vi "Initialize Andor.vi"() -> ()   [LabVIEW 2014]
uses:
  SubVIs/Initilize Globals.vi
  lib/Andorlib/atmcd32d.lvlib
panel:
  out "HS Speed":dbl format="%#_13g"
  out "Number HS Speeds":i32
  out "VS Speed":dbl format="%#_13g"
  out "Number VS Speeds":i32
  out "Camera FirmWare Version":i32
  out "Y-pixels":i32
  out "X-pixels":i32
  out "Error Out 2":errorcluster
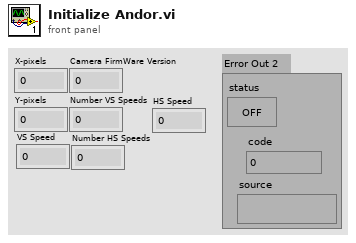
[diagram p1: front panel]
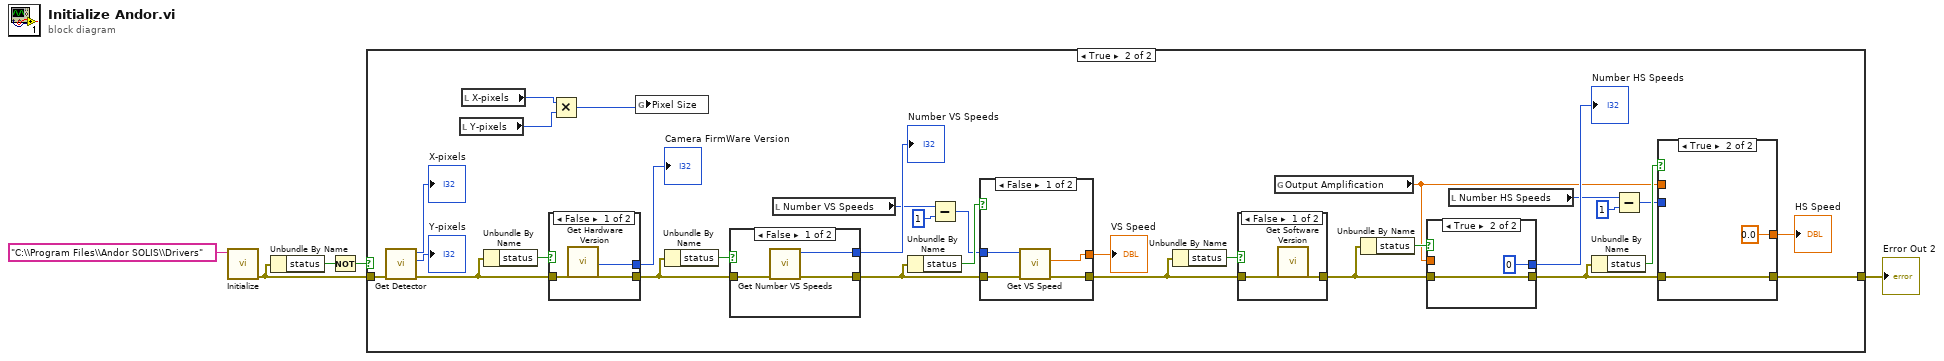
[diagram p0: block diagram]
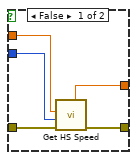
[diagram p3: hidden frame]
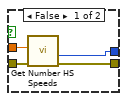
[diagram p4: hidden frame]
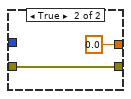
[diagram p6: hidden frame]
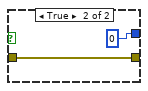
[diagram p7: hidden frame]
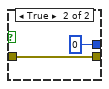
[diagram p8: hidden frame]
diagram:
  n1 = call "Initialize.vi"("dir"="C:\\Program Files\\Andor SOLIS\\Drivers") -> ("error out"=w2:errorcluster)  [unwired: 8 in, 2 out]
  n2 = Unbundle By Name(w2) -> ("status"=w5:bool)
  n3 = Not(x=w5) -> (.not. x?=w4:bool)
  n4 = case shown="True" w4 {
    tunnel: [w6 w25] -> w3
    tunnel: w2 -> [w6 w37]
    frame False {
    }
    frame True {
      n5 = call "Get Detector.vi"("error in (no error)"=w37) -> ("error out"=w30:errorcluster, "ypixels out"=→"Y-pixels":i32, "xpixels out"=→"X-pixels":i32)  [unwired: 7 in, 1 out]
      n6 = local read "Y-pixels"() -> (w8:i32)
      n7 = local read "X-pixels"() -> (w9:i32)
      n8 = Unbundle By Name(w30) -> ("status"=w36:bool)
      n9 = case shown="False" w36 {
        tunnel: w30 -> [w67 w69]
        tunnel: [w66 w69] -> w29
        tunnel: [w65 0] -> w21
        frame False {
          n10 = call "Get Hardware Version.vi"("error in (no error)"=w67) -> ("CameraFirmwareVersion out"=w65:u32, "error out"=w66:errorcluster)  [unwired: 19 in, 6 out]
        }
        frame True {
        }
      }
      "Camera FirmWare Version" <- w21
      n11 = Multiply(x=w9, y=w8) -> (x*y=w7:i32)
      n12 = global write "Initilize Globals.vi" "Pixel Size"(w7) -> ()
      n13 = Unbundle By Name(w29) -> ("status"=w35:bool)
      n14 = case shown="False" w35 {
        tunnel: w29 -> [w62 w64]
        tunnel: [w61 w64] -> w28
        tunnel: [w60 0] -> w20
        frame False {
          n15 = call "Get Number VS Speeds.vi"("error in (no error)"=w62) -> ("error out"=w61:errorcluster, "speeds out"=w60:i32)  [unwired: 8 in, 1 out]
        }
        frame True {
        }
      }
      "Number VS Speeds" <- w20
      n16 = local read "Number VS Speeds"() -> (w19:i32)
      n17 = Unbundle By Name(w28) -> ("status"=w34:bool)
      n18 = Subtract(x=w19, y=1) -> (x-y=w17:i32)
      n19 = case shown="False" w34 {
        tunnel: w28 -> [w56 w59]
        tunnel: [w57 w59] -> w27
        tunnel: w17 -> [w55 _]
        tunnel: [w54 0.0] -> w16
        frame False {
          n20 = call "Get VS Speed.vi"("error in (no error)"=w56, "index"=w55) -> ("error out"=w57:errorcluster, "speed out"=w54:sgl)  [unwired: 7 in, 1 out]
        }
        frame True {
        }
      }
      "VS Speed" <- w16
      n21 = Unbundle By Name(w27) -> ("status"=w33:bool)
      n22 = case shown="False" w33 {
        tunnel: w27 -> [w52 w53]
        tunnel: [w51 w53] -> w26
        frame False {
          n23 = call "Get Software Version.vi"("error in (no error)"=w52) -> ("error out"=w51:errorcluster)  [unwired: 19 in, 7 out]
        }
        frame True {
        }
      }
      n24 = global read "Initilize Globals.vi" "Output Amplification"() -> (w14:dbl)
      n25 = Unbundle By Name(w26) -> ("status"=w32:bool)
      n26 = case shown="True" w32 {
        tunnel: w26 -> [w48 w50]
        tunnel: [w47 w50] -> w24
        tunnel: w14 -> [w46 _]
        tunnel: [w45 0] -> w15
        frame False {
          n27 = call "Get Number HS Speeds.vi"("error in (no error)"=w48, "typ"=w46) -> ("error out"=w47:errorcluster, "speeds out"=w45:i32)  [unwired: 7 in, 1 out]
        }
        frame True {
        }
      }
      "Number HS Speeds" <- w15
      n28 = local read "Number HS Speeds"() -> (w13:i32)
      n29 = Unbundle By Name(w24) -> ("status"=w31:bool)
      n30 = Subtract(x=w13, y=1) -> (x-y=w11:i32)
      n31 = case shown="True" w31 {
        tunnel: w24 -> [w42 w44]
        tunnel: [w41 w44] -> w25
        tunnel: w14 -> [w40 _]
        tunnel: w11 -> [w39 _]
        tunnel: [w38 0.0] -> w10
        frame False {
          n32 = call "Get HS Speed.vi"("error in (no error)"=w42, "index"=w39, "typ"=w40) -> ("error out"=w41:errorcluster, "speed out"=w38:sgl)  [unwired: 6 in, 1 out]
        }
        frame True {
        }
      }
      "HS Speed" <- w10
    }
  }
  "Error Out 2" <- w3
